vi "SetZeroOffset.vi"(8 "Error in":errorcluster, 9 "ZeroOffset":dbl, 10 "Signal":refnum<k24>, 11 "DevicesAndSignals":T1) -> (0 "Error out":errorcluster, 3 "DevicesAndSignals":T1)   [LabVIEW 2016]
doc: "Sets the zero offset of the given analog in signal to the given value.\n\nSignal: Analog in signal whose zero offset should be set (notice that actually the channels zero offset will be set and therefore other signals that belong to the same channel are also affected).\nZeroOffset: Zero offset you want to use."
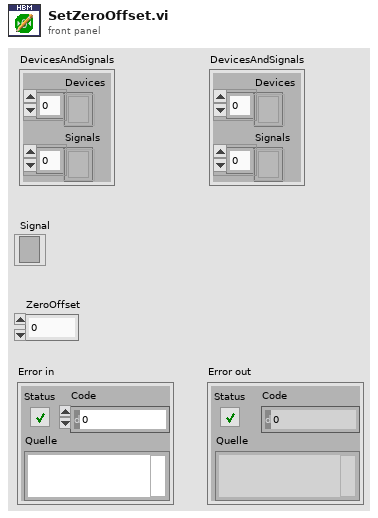
[diagram p1: front panel]
types:
  T1 = cluster{"Devices":refnum<k24>[], "Signals":refnum<k24>[]}
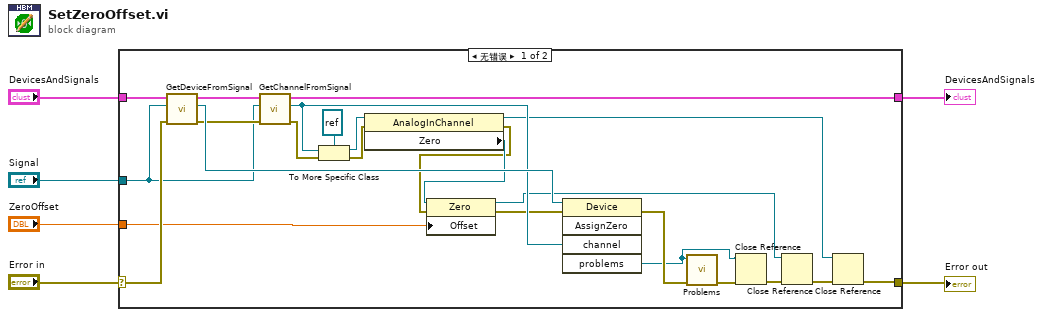
[diagram p0: block diagram]
diagram:
  n1 = case shown="无错误" "Error in" {
    selector: "Error in" -> [w26 w31]
    tunnel: "DevicesAndSignals" -> [w29 w30]
    tunnel: [w6 w31] -> w4
    tunnel: [w24 w30] -> _
    tunnel: "Signal" -> [w22 _]
    tunnel: "ZeroOffset" -> [w17 _]
    frame No Error {
      n2 = call "GetDeviceFromSignal.vi"("Error in"=w26, "Signal"=w22, "DevicesAndSignals"=w29) -> ("Error out"=w23:errorcluster, "Device"=w28:refnum<k24>, "DevicesAndSignals"=w25:T1)  [unwired: 6 in]
      n3 = call "GetChannelFromSignal.vi"("Error in"=w23, "Signal"=w22, "DevicesAndSignals"=w25) -> ("Error out"=w16:errorcluster, "Channel"=w21:refnum<k24>, "DevicesAndSignals"=w24:T1)  [unwired: 6 in]
      n4 = To More Specific Class(target class=refnum<k24> refnum ("Zielklasse"), reference=w21, error in=w16) -> (specific class reference=w19:refnum<k24>, error out=w15:errorcluster)
      n5 = property on="Eigenschaftsknoten" class="AnalogInChannel"(reference=w19, error in=w15) -> (reference out=w7:refnum<k24>, error out=w14:errorcluster, "Zero"=w18:refnum<k24>)
      n6 = property on="Eigenschaftsknoten" class="Zero"(reference=w18, error in=w14, "Offset"=w17) -> (reference out=w9:refnum<k24>, error out=w13:errorcluster)
      n7 = invoke on="Methodenknoten" class="Device" method="AssignZero"(reference=w28, error in=w13, "channel"=w21) -> (error out=w27:errorcluster, "problems"=w11:refnum<k24>)  [unwired: 2 in, 3 out]
      n8 = call "Problems.vi"("Error in"=w27, "Problems"=w11) -> ("Error out"=w12:errorcluster)  [unwired: 9 in]
      n9 = Close Reference(reference=w11, error in (no error)=w12) -> (error out=w10:errorcluster)
      n10 = Close Reference(reference=w9, error in (no error)=w10) -> (error out=w8:errorcluster)
      n11 = Close Reference(reference=w7, error in (no error)=w8) -> (error out=w6:errorcluster)
    }
    frame Error {
    }
  }
  "Error out" <- w4
  "DevicesAndSignals" <- "DevicesAndSignals"
